vi "ueye array to image.vi"(8 "Error In":errorcluster, 9 "Image In":T1, 10 "InArray":u8[](array[numeric]), 11 "Camera Reference":refnum<k24>) -> (0 "Error Out":errorcluster, 1 "Image Out":T1, 3 "Camera Reference Out":refnum<k24>)   [LabVIEW 2017, in "Vision.lvlib"]
doc: "ArrayToVision converts 24/32-bit one-dimensional arrays to a two-dimensional U32 array."
uses:
  Vision.lvlib
  C:/Users/Caleb/Desktop/nebraska-silicon-lab/pixel-gantry-extra/LV/bin/uEyeDotNet.dll
  bin/uEyeDotNet.dll
  <vilib>/vision/Image Controls.llb/IMAQ Image.ctl
panel:
  # "Output"
  # "Input"
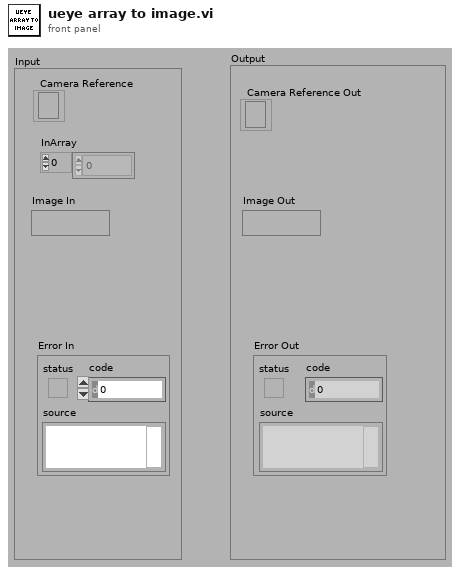
[diagram p1: front panel]
types:
  T1 = typedef "IMAQ Image.ctl" = refnum<image>
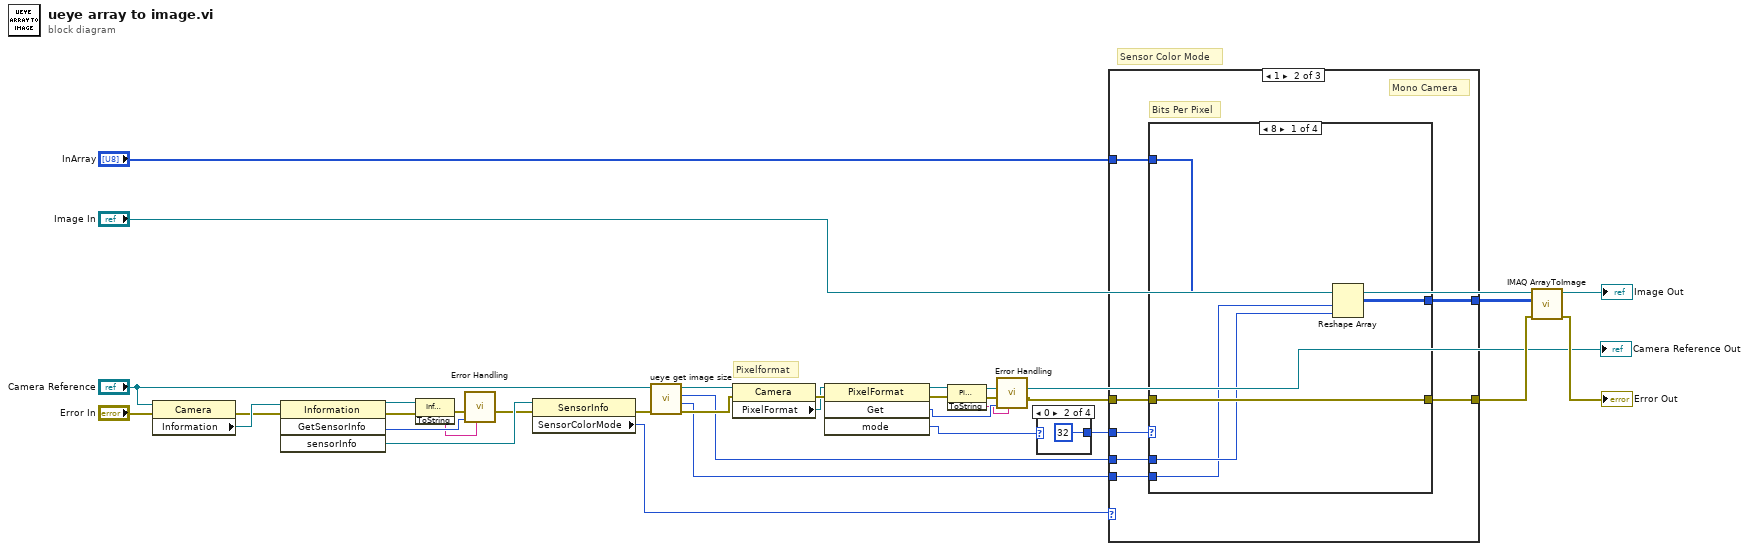
[diagram p0: block diagram]
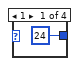
[diagram p2: hidden frame]
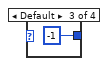
[diagram p3: hidden frame]
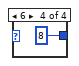
[diagram p4: hidden frame]
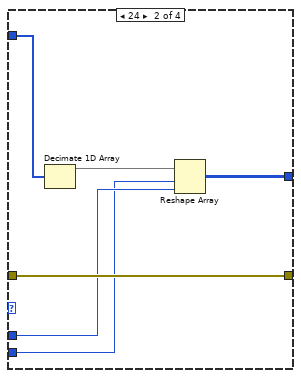
[diagram p6: hidden frame]
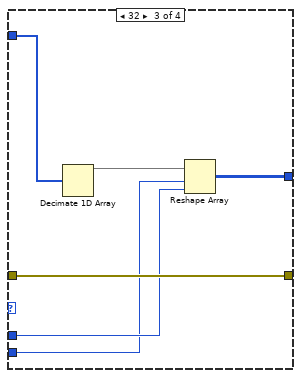
[diagram p7: hidden frame]
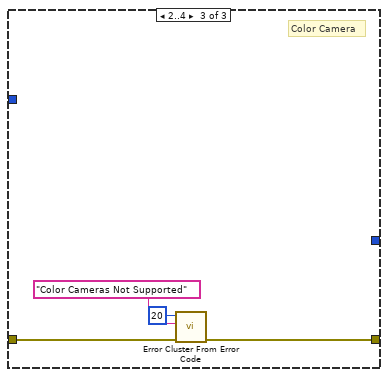
[diagram p9: hidden frame]
diagram:
  # "Sensor Color Mode"
  # "Pixelformat"
  n1 = property on="Eigenschaftsknoten" class="Camera"(reference="Camera Reference", error in="Error In") -> (error out=w31:errorcluster, "Information"=w34:refnum<k24>)  [unwired: 1 out]
  n2 = invoke class="Information" method="GetSensorInfo"(reference=w34, error in=w31) -> (reference out=w28:refnum<k24>, error out=w27:errorcluster, "GetSensorInfo"=w19:i32, "sensorInfo"=w33:refnum<k24>)  [unwired: 2 in]
  n3 = invoke class="Information" method="ToString"(reference=w28, error in=w27) -> (error out=w20:errorcluster, "ToString"=w18:string)  [unwired: 1 in, 1 out]
  n4 = call "Error Handling.vi"("Error String"=w18, "Error Code"=w19, "Error In"=w20) -> ("Error Out"=w17:errorcluster)  [unwired: 8 in]
  n5 = property class="SensorInfo"(reference=w33, error in=w17) -> (error out=w14:errorcluster, "SensorColorMode"=w32:i32)  [unwired: 1 out]
  n6 = call "ueye get image size.vi"("Error In"=w14, ".NET (Reference)"="Camera Reference") -> ("Error Out"=w13:errorcluster, "Height"=w11:i32, "Width"=w12:i32, ".NET (Reference)"=w15:refnum<k24>)  [unwired: 6 in]
  n7 = property class="Camera"(reference=w15, error in=w13) -> (error out=w24:errorcluster, "PixelFormat"=w23:refnum<k24>)  [unwired: 1 out]
  n8 = invoke class="PixelFormat" method="Get"(reference=w23, error in=w24) -> (reference out=w26:refnum<k24>, error out=w25:errorcluster, "Get"=w8:i32, "mode"=w22:i32)  [unwired: 2 in]
  n9 = invoke class="PixelFormat" method="ToString"(reference=w26, error in=w25) -> (reference out=→"Camera Reference Out":refnum<k24>, error out=w10:errorcluster, "ToString"=w7:string)  [unwired: 1 in]
  n10 = call "Error Handling.vi"("Error String"=w7, "Error Code"=w8, "Error In"=w10) -> ("Error Out"=w9:errorcluster)  [unwired: 8 in]
  n11 = case shown="0" w22 {
    tunnel: [24 32 -1 8] -> w21
    frame 1 {
    }
    frame 0 {
    }
    frame Default {
    }
    frame 6 {
    }
  }
  n12 = case shown="1" w32 {
    tunnel: "InArray" -> [_ w44 _]
    tunnel: w12 -> [_ w42 _]
    tunnel: w11 -> [_ w41 _]
    tunnel: w21 -> [_ w43 _]
    tunnel: w9 -> [w39 w46 w67]
    tunnel: [w39 w45 w68] -> w5
    tunnel: [_ w40 _] -> w6
    frame 0, Default {
    }
    frame 1 {
      # "Bits Per Pixel"
      # "Mono Camera"
      n13 = case shown="8" w43 {
        tunnel: w44 -> [w47 w57 w62 _]
        tunnel: w41 -> [w48 w53 w59 _]
        tunnel: w42 -> [w49 w54 w60 _]
        tunnel: [w51 w56 w63 _] -> w40
        tunnel: w46 -> [w50 w55 w61 w64]
        tunnel: [w50 w55 w61 w64] -> w45
        frame 8 {
          n14 = Reshape Array(w47, w48, w49) -> (w51:u8[][])
        }
        frame 24 {
          n15 = Decimate 1D Array(w57) -> (w52:u8[])  [unwired: 2 out]
          n16 = Reshape Array(w52, w53, w54) -> (w56:u8[][])
        }
        frame 32 {
          n17 = Decimate 1D Array(w62) -> (w58:u8[])  [unwired: 3 out]
          n18 = Reshape Array(w58, w59, w60) -> (w63:u8[][])
        }
        frame Default {
        }
      }
    }
    frame 2..4 {
      # "Color Camera"
      n19 = call <vilib>:"Error Cluster From Error Code.vi"("error in (no error)"=w67, "error message (\"\")"="Color Cameras Not Supported" ("error message (\"\")"), "error code (0)"=20) -> ("error out"=w68:errorcluster)  [unwired: 6 in]
    }
  }
  n20 = call "IMAQ ArrayToImage"("error in (no error)"=w5, "Image Pixels (U8)"=w6, "Image"="Image In") -> ("error out"=→"Error Out":errorcluster, "Image Out"=→"Image Out":T1)  [unwired: 7 in]
